vi "rszvl_core_global.vi"() -> ()   [LabVIEW 2014] (continued)
Callback"="", "Coerce Callback"="", "User Callback"="", "Supported Models"="", "Instrument Options"="", "Repeated Capabilities"="", "Restricted Repeated Capabilities"="", "Help"="This attribute defines an absolute threshold value for limit lines with relative Y axis scaling. The absolute threshold value is used in the limit check as soon as it exceeds the relative limit value.\n\nAvailable Repeated Capabilities:\nLimit: L1,L2,L3,L4,L5,L6,L7,L8\r\n\nRemote-control command(s):\nCALCulate<1|2>:LIMit<1 to 8>:LOWer:THReshold", "Flags"={"OPC Wait"=FALSE, "Dont check status"=FALSE, "*WAI"=FALSE}, "Check Status Callback"=""}, {"Level"=3, "Descriptive Name"="Limit Line Lower Offset", "Class Only"=FALSE, "Data Type"=1, "Access"=2, "Identifier"="RSZVL_LIMIT_LOWER_OFFSET", "Range Table"="rszvl_rngRefLevel", "Command"="CALC:LIM{Limit}:LOW:OFFS", "Read Callback"="", "Write Callback"="", "Range Callback"="", "Check Callback"="", "Rngtable Callback"="", "Coerce Callback"="", "User Callback"="", "Supported Models"="", "Instrument Options"="", "Repeated Capabilities"="", "Restricted Repeated Capabilities"="", "Help"="This attribute defines an offset for the Y axis of the selected relative lower limit line. In contrast to SHIF, the line is not shifted by modifying the individual Y values but by means of an additive offset.\n\nAvailable Repeated Capabilities:\nLimit: L1,L2,L3,L4,L5,L6,L7,L8\r\n\nRemote-control command(s):\nCALCulate<1|2>:LIMit<1 to 8>:LOWer:OFFSet", "Flags"={"OPC Wait"=FALSE, "Dont check status"=FALSE, "*WAI"=FALSE}, "Check Status Callback"=""}, {"Level"=3, "Descriptive Name"="Limit Line Lower Shift", "Class Only"=FALSE, "Data Type"=1, "Access"=1, "Identifier"="RSZVL_LIMIT_LOWER_SHIFT", "Range Table"="rszvl_rngLimitOffset", "Command"="CALC:LIM{Limit}:LOW:SHIF", "Read Callback"="", "Write Callback"="", "Range Callback"="", "Check Callback"="", "Rngtable Callback"="", "Coerce Callback"="", "User Callback"="", "Supported Models"="", "Instrument Options"="", "Repeated Capabilities"="", "Restricted Repeated Capabilities"="", "Help"="This attribute shifts a limit line by the indicated value in Y direction. In contrast to offset, the line is shifted by modifying the individual Y values but not by means of an additive offset.\n\nAvailable Repeated Capabilities:\nLimit: L1,L2,L3,L4,L5,L6,L7,L8\r\n\nRemote-control command(s):\nCALCulate<1|2>:LIMit<1 to 8>:LOWer:SHIFt", "Flags"={"OPC Wait"=FALSE, "Dont check status"=FALSE, "*WAI"=FALSE}, "Check Status Callback"=""}, {"Level"=2, "Descriptive Name"="Upper Limit", "Class Only"=TRUE, "Data Type"=0, "Access"=0, "Identifier"="", "Range Table"="", "Command"="", "Read Callback"="", "Write Callback"="", "Range Callback"="", "Check Callback"="", "Rngtable Callback"="", "Coerce Callback"="", "User Callback"="", "Supported Models"="", "Instrument Options"="", "Repeated Capabilities"="", "Restricted Repeated Capabilities"="", "Help"="(1) Limit Line Upper State:\nThis attribute switches on or off the indicated limit line.\n\n(2) Limit Line Upper Scaling:\nThis command selects the relative or absolute scaling for the Y axis of the selected upper limit line. Selecting RELative causes the unit to be switched to DB.\n\n(3) Limit Line Upper Spacing:\nThis attribute selects linear or logarithmic interpolation for the upper limit line.\n\n(4) Limit Line Upper Margin:\nThis attribute defines a margin to an upper limit line, at which out-of-limit values are signalled (if the limit check is active), but not handled as a violation of the limit value.\n\n(5) Limit Line Upper Threshold:\nThis attribute defines an absolute threshold value for limit lines with relative Y axis scaling. The absolute threshold value is used in the limit check as soon as it exceeds the relative limit value.\n\n(6) Limit Line Upper Offset:\nThis attribute defines an offset for the Y axis of the selected relative upper limit line. In contrast to shift, the line is not shifted by modifying the individual Y values but by means of an additive offset.\n\n(7) Limit Line Upper Shift:\nThis attribute moves a limit line by the indicated value in Y direction. In contrast to offset, the line is shifted by modifying the individual Y values and not by means of an additive offset.", "Flags"={"OPC Wait"=FALSE, "Dont check status"=FALSE, "*WAI"=FALSE}, "Check Status Callback"=""}, {"Level"=3, "Descriptive Name"="Limit Line Upper State", "Class Only"=FALSE, "Data Type"=3, "Access"=2, "Identifier"="RSZVL_LIMIT_UPPER_STATE", "Range Table"="", "Command"="CALC:LIM{Limit}:UPP:STAT", "Read Callback"="", "Write Callback"="", "Range Callback"="", "Check Callback"="", "Rngtable Callback"="", "Coerce Callback"="", "User Callback"="", "Supported Models"="", "Instrument Options"="", "Repeated Capabilities"="", "Restricted Repeated Capabilities"="", "Help"="This attribute switches on or off the indicated limit line.\n\nAvailable Repeated Capabilities:\nLimit: L1,L2,L3,L4,L5,L6,L7,L8\r\n\nRemote-control command(s):\nCALCulate<1|2>:LIMit<1 to 8>:UPPer:STATe ON | OFF", "Flags"={"OPC Wait"=FALSE, "Dont check status"=FALSE, "*WAI"=FALSE}, "Check Status Callback"=""}, {"Level"=3, "Descriptive Name"="Limit Line Upper Scaling", "Class Only"=FALSE, "Data Type"=0, "Access"=2, "Identifier"="RSZVL_LIMIT_UPPER_SCALING", "Range Table"="rszvl_rngAbsRel", "Command"="CALC:LIM{Limit}:UPP:MODE", "Read Callback"="", "Write Callback"="", "Range Callback"="", "Check Callback"="", "Rngtable Callback"="", "Coerce Callback"="", "User Callback"="", "Supported Models"="", "Instrument Options"="", "Repeated Capabilities"="", "Restricted Repeated Capabilities"="", "Help"="This command selects the relative or absolute scaling for the Y axis of the selected upper limit line. Selecting RELative causes the unit to be switched to DB.\n\nAvailable Repeated Capabilities:\nLimit: L1,L2,L3,L4,L5,L6,L7,L8\r\n\nRemote-control command(s):\nCALCulate<1|2>:LIMit<1 to 8>:UPPer:MODE RELative | ABSolute", "Flags"={"OPC Wait"=FALSE, "Dont check status"=FALSE, "*WAI"=FALSE}, "Check Status Callback"=""}, {"Level"=3, "Descriptive Name"="Limit Line Upper Spacing", "Class Only"=FALSE, "Data Type"=0, "Access"=2, "Identifier"="RSZVL_LIMIT_UPPER_SPACING", "Range Table"="rszvl_rngLinLog", "Command"="CALC:LIM{Limit}:UPP:SPAC", "Read Callback"="", "Write Callback"="", "Range Callback"="", "Check Callback"="", "Rngtable Callback"="", "Coerce Callback"="", "User Callback"="", "Supported Models"="", "Instrument Options"="", "Repeated Capabilities"="", "Restricted Repeated Capabilities"="", "Help"="This attribute selects linear or logarithmic interpolation for the upper limit line.\n\nAvailable Repeated Capabilities:\nLimit: L1,L2,L3,L4,L5,L6,L7,L8\r\n\nRemote-control command(s):\nCALCulate<1|2>:LIMit<1 to 8>:UPPer:SPACing LINear | LOGarithmic", "Flags"={"OPC Wait"=FALSE, "Dont check status"=FALSE, "*WAI"=FALSE}, "Check Status Callback"=""}, {"Level"=3, "Descriptive Name"="Limit Line Upper Margin", "Class Only"=FALSE, "Data Type"=1, "Access"=2, "Identifier"="RSZVL_LIMIT_UPPER_MARGIN", "Range Table"="rszvl_rngLimitMargin", "Command"="CALC:LIM{Limit}:UPP:MARG", "Read Callback"="", "Write Callback"="", "Range Callback"="", "Check Callback"="", "Rngtable Callback"="", "Coerce Callback"="", "User Callback"="", "Supported Models"="", "Instrument Options"="", "Repeated Capabilities"="", "Restricted Repeated Capabilities"="", "Help"="This attribute defines a margin to an upper limit line, at which out-of-limit values are signalled (if the limit check is active), but not handled as a violation of the limit value.\n\nAvailable Repeated Capabilities:\nLimit: L1,L2,L3,L4,L5,L6,L7,L8\r\n\nRemote-control command(s):\nCALCulate<1|2>:LIMit<1 to 8>:UPPer:MARGin", "Flags"={"OPC Wait"=FALSE, "Dont check status"=FALSE, "*WAI"=FALSE}, "Check Status Callback"=""}, {"Level"=3, "Descriptive Name"="Limit Line Upper Threshold", "Class Only"=FALSE, "Data Type"=1, "Access"=2, "Identifier"="RSZVL_LIMIT_UPPER_THRESHOLD", "Range Table"="rszvl_rngRefLevel", "Command"="CALC:LIM{Limit}:UPP:THR", "Read Callback"="", "Write Callback"="", "Range Callback"="", "Check Callback"="", "Rngtable Callback"="", "Coerce Callback"="", "User Callback"="", "Supported Models"="", "Instrument Options"="", "Repeated Capabilities"="", "Restricted Repeated Capabilities"="", "Help"="This attribute defines an absolute threshold value for limit lines with relative Y axis scaling. The absolute threshold value is used in the limit check as soon as it exceeds the relative limit value.\n\nAvailable Repeated Capabilities:\nLimit: L1,L2,L3,L4,L5,L6,L7,L8\r\n\nRemote-control command(s):\nCALCulate<1|2>:LIMit<1 to 8>:UPPer:THReshold", "Flags"={"OPC Wait"=FALSE, "Dont check status"=FALSE, "*WAI"=FALSE}, "Check Status Callback"=""}, {"Level"=3, "Descriptive Name"="Limit Line Upper Offset", "Class Only"=FALSE, "Data Type"=1, "Access"=2, "Identifier"="RSZVL_LIMIT_UPPER_OFFSET", "Range Table"="rszvl_rngRefLevel", "Command"="CALC:LIM{Limit}:UPP:OFFS", "Read Callback"="", "Write Callback"="", "Range Callback"="", "Check Callback"="", "Rngtable Callback"="", "Coerce Callback"="", "User Callback"="", "Supported Models"="", "Instrument Options"="", "Repeated Capabilities"="", "Restricted Repeated Capabilities"="", "Help"="This attribute defines an offset for the Y axis of the selected relative upper limit line. In contrast to shift, the line is not shifted by modifying the individual Y values but by means of an additive offset.\n\nAvailable Repeated Capabilities:\nLimit: L1,L2,L3,L4,L5,L6,L7,L8\r\n\nRemote-control command(s):\nCALCulate<1|2>:LIMit<1 to 8>:UPPer:OFFSet", "Flags"={"OPC Wait"=FALSE, "Dont check status"=FALSE, "*WAI"=FALSE}, "Check Status Callback"=""}, {"Level"=3, "Descriptive Name"="Limit Line Upper Shift", "Class Only"=FALSE, "Data Type"=1, "Access"=1, "Identifier"="RSZVL_LIMIT_UPPER_SHIFT", "Range Table"="rszvl_rngLimitOffset", "Command"="CALC:LIM{Limit}:UPP:SHIF", "Read Callback"="", "Write Callback"="", "Range Callback"="", "Check Callback"="", "Rngtable Callback"="", "Coerce Callback"="", "User Callback"="", "Supported Models"="", "Instrument Options"="", "Repeated Capabilities"="", "Restricted Repeated Capabilities"="", "Help"="This attribute moves a limit line by the indicated value in Y direction. In contrast to offset, the line is shifted by modifying the individual Y values and not by means of an additive offset.\n\nAvailable Repeated Capabilities:\nLimit: L1,L2,L3,L4,L5,L6,L7,L8\r\n\nRemote-control command(s):\nCALCulate<1|2>:LIMit<1 to 8>:UPPer:SHIFt", "Flags"={"OPC Wait"=FALSE, "Dont check status"=FALSE, "*WAI"=FALSE}, "Check Status Callback"=""}, {"Level"=2, "Descriptive Name"="Display Lines", "Class Only"=TRUE, "Data Type"=0, "Access"=0, "Identifier"="", "Range Table"="", "Command"="", "Read Callback"="", "Write Callback"="", "Range Callback"="", "Check Callback"="", "Rngtable Callback"="", "Coerce Callback"="", "User Callback"="", "Supported Models"="", "Instrument Options"="", "Repeated Capabilities"="", "Restricted Repeated Capabilities"="", "Help"="(1) Threshold Line State:\nThis attribute switches on or off the threshold line.\n\n(2) Threshold Line Position:\nThis attribute defines the threshold value for the maximum/minimum search of markers with marker search functions MAX PEAK, NEXT PEAK, etc.\n\n(3) Display Line State:\nThis attribute switches Display Line 1 or 2 (level lines) on or off.\n\n(4) Display Line Position:\nThis attribute defines the position of Display Line 1 or 2. These lines enable the user to mark any levels in the diagram. The unit depends on the setting made with CALC:UNIT.\n\n(5) Frequency Line State:\nThis attribute switches the frequency line on or off.\n\n(6) Frequency Line Position:\nThis attribute defines the position of the frequency lines.\nThe frequency lines mark the frequencies. Frequency lines are only available with SPAN > 0.\n\n(7) Time Line State:\nThis attribute switches the time line on or off.\n\n(8) Time Line Position:\nThis attribute defines the position of the time lines.\nThe time lines mark the times. Time lines are only available with SPAN = 0.", "Flags"={"OPC Wait"=FALSE, "Dont check status"=FALSE, "*WAI"=FALSE}, "Check Status Callback"=""}, {"Level"=3, "Descriptive Name"="Threshold Line State", "Class Only"=FALSE, "Data Type"=3, "Access"=2, "Identifier"="RSZVL_ATTR_THRLINE_STATE", "Range Table"="", "Command"="CALC:THR:STAT", "Read Callback"="", "Write Callback"="", "Range Callback"="", "Check Callback"="", "Rngtable Callback"="", "Coerce Callback"="", "User Callback"="", "Supported Models"="", "Instrument Options"="", "Repeated Capabilities"="", "Restricted Repeated Capabilities"="", "Help"="This attribute switches on or off the threshold line.\n\nAvailable Repeated Capabilities:\nNone\n\nRemote-control command(s):\nCALCulate<1|2>:THReshold:STATe ON | OFF", "Flags"={"OPC Wait"=FALSE, "Dont check status"=FALSE, "*WAI"=FALSE}, "Check Status Callback"=""}, {"Level"=3, "Descriptive Name"="Threshold Line Position", "Class Only"=FALSE, "Data Type"=1, "Access"=2, "Identifier"="RSZVL_ATTR_THRLINE_POSITION", "Range Table"="", "Command"="CALC:THR", "Read Callback"="", "Write Callback"="", "Range Callback"="", "Check Callback"="", "Rngtable Callback"="", "Coerce Callback"="", "User Callback"="", "Supported Models"="", "Instrument Options"="", "Repeated Capabilities"="", "Restricted Repeated Capabilities"="", "Help"="This attribute defines the threshold value for the maximum/minimum search of markers with marker search functions MAX PEAK, NEXT PEAK, etc.\n\nAvailable Repeated Capabilities:\nNone\n\nRemote-control command(s):\nCALCulate<1|2>:THReshold", "Flags"={"OPC Wait"=FALSE, "Dont check status"=FALSE, "*WAI"=FALSE}, "Check Status Callback"=""}, {"Level"=3, "Descriptive Name"="Display Line State", "Class Only"=FALSE, "Data Type"=3, "Access"=2, "Identifier"="RSZVL_ATTR_DLINE_STATE", "Range Table"="", "Command"="CALC:DLIN{Line}:STAT", "Read Callback"="", "Write Callback"="", "Range Callback"="", "Check Callback"="", "Rngtable Callback"="", "Coerce Callback"="", "User Callback"="", "Supported Models"="", "Instrument Options"="", "Repeated Capabilities"="", "Restricted Repeated Capabilities"="", "Help"="This attribute switches Display Line 1 or 2 (level lines) on or off.\n\nAvailable Repeated Capabilities:\nLine: L1,L2\r\n\nRemote-control command(s):\nCALCulate<1|2>:DLINe<1|2>:STATe ON | OFF", "Flags"={"OPC Wait"=FALSE, "Dont check status"=FALSE, "*WAI"=FALSE}, "Check Status Callback"=""}, {"Level"=3, "Descriptive Name"="Display Line Position", "Class Only"=FALSE, "Data Type"=1, "Access"=2, "Identifier"="RSZVL_ATTR_DLINE_POSITION", "Range Table"="", "Command"="CALC:DLIN{Line}", "Read Callback"="", "Write Callback"="", "Range Callback"="", "Check Callback"="", "Rngtable Callback"="", "Coerce Callback"="", "User Callback"="", "Supported Models"="", "Instrument Options"="", "Repeated Capabilities"="", "Restricted Repeated Capabilities"="", "Help"="This attribute defines the position of Display Line 1 or 2. These lines enable the user to mark any levels in the diagram. The unit depends on the setting made with CALC:UNIT.\n\nAvailable Repeated Capabilities:\nLine: L1,L2\r\n\nRemote-control command(s):\nCALCulate<1|2>:DLINe<1|2>", "Flags"={"OPC Wait"=FALSE, "Dont check status"=FALSE, "*WAI"=FALSE}, "Check Status Callback"=""}, {"Level"=3, "Descriptive Name"="Frequency Line State", "Class Only"=FALSE, "Data Type"=3, "Access"=2, "Identifier"="RSZVL_ATTR_FLINE_STATE", "Range Table"="", "Command"="CALC:FLIN{Line}:STAT", "Read Callback"="", "Write Callback"="", "Range Callback"="", "Check Callback"="", "Rngtable Callback"="", "Coerce Callback"="", "User Callback"="", "Supported Models"="", "Instrument Options"="", "Repeated Capabilities"="", "Restricted Repeated Capabilities"="", "Help"="This attribute switches the frequency line on or off.\n\nAvailable Repeated Capabilities:\nLine: L1,L2\r\n\nRemote-control command(s):\nCALCulate<1|2>:FLINe<1|2>:STATe ON | OFF", "Flags"={"OPC Wait"=FALSE, "Dont check status"=FALSE, "*WAI"=FALSE}, "Check Status Callback"=""}, {"Level"=3, "Descriptive Name"="Frequency Line Position", "Class Only"=FALSE, "Data Type"=1, "Access"=2, "Identifier"="RSZVL_ATTR_FLINE_POSITION", "Range Table"="", "Command"="CALC:FLIN{Line}", "Read Callback"="", "Write Callback"="", "Range Callback"="", "Check Callback"="", "Rngtable Callback"="", "Coerce Callback"="", "User Callback"="", "Supported Models"="", "Instrument Options"="", "Repeated Capabilities"="", "Restricted Repeated Capabilities"="", "Help"="This attribute defines the position of the frequency lines.\nThe frequency lines mark the frequencies. Frequency lines are only available with SPAN > 0.\n\nAvailable Repeated Capabilities:\nLine: L1,L2\r\n\nRemote-control command(s):\nCALCulate<1|2>:FLINe<1|2>", "Flags"={"OPC Wait"=FALSE, "Dont check status"=FALSE, "*WAI"=FALSE}, "Check Status Callback"=""}, {"Level"=3, "Descriptive Name"="Time Line State", "Class Only"=FALSE, "Data Type"=3, "Access"=2, "Identifier"="RSZVL_ATTR_TLINE_STATE", "Range Table"="", "Command"="CALC:TLIN{Line}:STAT", "Read Callback"="", "Write Callback"="", "Range Callback"="", "Check Callback"="", "Rngtable Callback"="", "Coerce Callback"="", "User Callback"="", "Supported Models"="", "Instrument Options"="", "Repeated Capabilities"="", "Restricted Repeated Capabilities"="", "Help"="This attribute switches the time line on or off.\n\nAvailable Repeated Capabilities:\nLine: L1,L2\r\n\nRemote-control command(s):\nCALCulate<1|2>:TLINe<1|2>:STATe ON | OFF", "Flags"={"OPC Wait"=FALSE, "Dont check status"=FALSE, "*WAI"=FALSE}, "Check Status Callback"=""}, {"Level"=3, "Descriptive Name"="Time Line Position", "Class Only"=FALSE, "Data Type"=1, "Access"=2, "Identifier"="RSZVL_ATTR_TLINE_POSITION", "Range Table"="rszvl_rngTimeLinePos", "Command"="CALC:TLIN{Line}", "Read Callback"="", "Write Callback"="", "Range Callback"="", "Check Callback"="", "Rngtable Callback"="", "Coerce Callback"="", "User Callback"="", "Supported Models"="", "Instrument Options"="", "Repeated Capabilities"="", "Restricted Repeated Capabilities"="", "Help"="This attribute defines the position of the time lines.\nThe time lines mark the times. Time lines are only available with SPAN = 0.\n\nAvailable Repeated Capabilities:\nLine: L1,L2\r\n\nRemote-control command(s):\nCALCulate<1|2>:TLINe<1|2>", "Flags"={"OPC Wait"=FALSE, "Dont check status"=FALSE, "*WAI"=FALSE}, "Check Status Callback"=""}, {"Level"=1, "Descriptive Name"="Trigger", "Class Only"=TRUE, "Data Type"=0, "Access"=0, "Identifier"="", "Range Table"="", "Command"="", "Read Callback"="", "Write Callback"="", "Range Callback"="", "Check Callback"="", "Rngtable Callback"="", "Coerce Callback"="", "User Callback"="", "Supported Models"="", "Instrument Options"="", "Repeated Capabilities"="", "Restricted Repeated Capabilities"="", "Help"="(1) Trigger Source:\nThis attribute selects the trigger source for the start of a sweep.\n\n(2) Trigger Delay:\nThis attribute defines the length of the trigger delay.\n\nNote:\n(1) A negative delay time (pretrigger) can be set in the time domain (span < 0 Hz) only.\n\n(3) Trigger Slope:\nThis attribute selects the slope of the trigger signal. The selected trigger slope applies to all trigger signal sources .\n\n(4) External Trigger (Class):\nAttributes to configure and control external triggers.\n\n(1) External Gate:\nThis attribute switches on/off the sweep control by an external gate signal. If the external gate is selected the trigger source is automatically switched to EXTernal as well. \nIn case of measurement with external gate, the measured values are recorded as long as the gate is opened. There are two possibilities:\n\n1. The gate is edge-triggered (SWEep:EGATe:TYPE EDGE): After detection of the set gate signal edge, the gate remains open until the gate delay (SWEep:EGATe:HOLDoff) has expired.\n\n2. The gate is level-triggered (SWEep:EGATe:TYPE LEVel): After detection of the gate signal, the gate remains open until the gate signal disappears.\n\nA delay between applying the gate signal and the start of recording measured values can be defined\nwith SWEep:EGATe:HOLDoff.\nDuring a sweep the gate can be opened and closed several times. The synchronization mechanisms\nwith *OPC, *OPC? and *WAI remain completely unaffected.\nThe sweep end is detected when the required number of measurement points (625 in analyzer\nmode) has been recorded.\n\nNote: \n(1) This attribute is not available for GSM/EDGE measurements modulation accuracy (MAC),\nphase/frequency error (PFE), power versus time (PVT ), carrier power (CPW), spectrum\ndue to switching (TRA) and spurious emissions (SPU).\n\n(2) External Gate Delay:\nThis attribute defines the delay time between the external gate signal and the continuation of the sweep.\n\n(3) External Gate Mode:\nThis attribute sets the type of triggering (level or edge) by the external gate signal.\nThe gate opening time cannot be defined with the parameter EGATe:LENGth in case of level triggering. The gate is closed when the gate signal disappears.\n\n(4) External Gate Polarity:\nThis attribute determines the polarity of the external gate signal. The setting is valid both for the edge of an edge-triggered signal and the level of a level-triggered signal.\n\n(5) External Gate Length:\nThis attribute determines the time interval during which the instrument sweeps.\n\n(6) External Gate Signal Source:\nThis attribute toggles between external gate signal and IF power signal as a signal source for the gate mode. If an IF power signal is used, the gate is opened as soon as a signal at > -20 dBm is detected within the IF path bandwidth (50 MHz).\n\n\n\n(5) Video Trigger (Class):\nAttributes to configure and control video triggers.\n\n(1) Video Trigger Level:\nThis attribute sets the level of the video trigger source.\n\n\n\n(6) IF Power Trigger (Class):\nIF Power Trigger configuration.\n\n(1) Trigger IF Power Level:\nThis attribute sets the level of the IF power trigger source.\n\n(2) Trigger IF Power Offset:\nThis attribute sets the holding time before the next IF power trigger event.\n\n(3) Trigger IF Power Hysteresis:\nThis attribute sets the limit that the hysteresis value has to fall below in order to trigger the next measurement.\n\n\n\n(7) Time Trigger (Class):\nTime Trigger configuration.\n\n(1) Time Interval:\nThis attribute sets the time intervall for the time trigger source.", "Flags"={"OPC Wait"=FALSE, "Dont check status"=FALSE, "*WAI"=FALSE}, "Check Status Callback"=""}, {"Level"=2, "Descriptive Name"="Trigger Source", "Class Only"=FALSE, "Data Type"=0, "Access"=2, "Identifier"="RSZVL_ATTR_TRIGGER_SOURCE", "Range Table"="rszvl_rngTriggerSource", "Command"="TRIG{Channel}:SOUR", "Read Callback"="", "Write Callback"="", "Range Callback"="", "Check Callback"="", "Rngtable Callback"="", "Coerce Callback"="", "User Callback"="", "Supported Models"="", "Instrument Options"="", "Repeated Capabilities"="", "Restricted Repeated Capabilities"="", "Help"="This attribute selects the trigger source for the start of a sweep.\n\nAvailable Repeated Capabilities:\nChannel: CH1,CH2,CH3,CH4,CH5,CH6,CH7,CH8,CH9,CH10,CH11,CH12,CH13,CH14,CH15,CH16,CH17,CH18,CH19,CH20\r\n\nRemote-control command(s):\nTRIGger<Channel>[:SEQuence]:SOURce", "Flags"={"OPC Wait"=FALSE, "Dont check status"=FALSE, "*WAI"=FALSE}, "Check Status Callback"=""}, {"Level"=2, "Descriptive Name"="Trigger Delay", "Class Only"=FALSE, "Data Type"=1, "Access"=2, "Identifier"="RSZVL_ATTR_TRIGGER_DELAY", "Range Table"="rszvl_rngTriggerDelay", "Command"="TRIG{Channel}:HOLD", "Read Callback"="", "Write Callback"="", "Range Callback"="", "Check Callback"="", "Rngtable Callback"="", "Coerce Callback"="", "User Callback"="", "Supported Models"="", "Instrument Options"="", "Repeated Capabilities"="", "Restricted Repeated Capabilities"="", "Help"="This attribute defines the length of the trigger delay.\n\nNote:\n(1) A negative delay time (pretrigger) can be set in the time domain (span < 0 Hz) only.\n\nAvailable Repeated Capabilities:\nChannel: CH1,CH2,CH3,CH4,CH5,CH6,CH7,CH8,CH9,CH10,CH11,CH12,CH13,CH14,CH15,CH16,CH17,CH18,CH19,CH20\r\n\nRemote-control command(s):\nTRIGger<Channel>[:SEQuence]:HOLDoff", "Flags"={"OPC Wait"=FALSE, "Dont check status"=FALSE, "*WAI"=FALSE}, "Check Status Callback"=""}, {"Level"=2, "Descriptive Name"="Trigger Slope", "Class Only"=FALSE, "Data Type"=0, "Access"=2, "Identifier"="RSZVL_ATTR_TRIGGER_SLOPE", "Range Table"="rszvl_rngPolarity", "Command"="TRIG{Channel}:SLOP", "Read Callback"="", "Write Callback"="", "Range Callback"="", "Check Callback"="", "Rngtable Callback"="", "Coerce Callback"="", "User Callback"="", "Supported Models"="", "Instrument Options"="", "Repeated Capabilities"="", "Restricted Repeated Capabilities"="", "Help"="This attribute selects the slope of the trigger signal. The selected trigger slope applies to all trigger signal sources .\n\nAvailable Repeated Capabilities:\nChannel: CH1,CH2,CH3,CH4,CH5,CH6,CH7,CH8,CH9,CH10,CH11,CH12,CH13,CH14,CH15,CH16,CH17,CH18,CH19,CH20\r\n\nRemote-control command(s):\nTRIGger<Channel>[:SEQuence]:SLOPe POSitive | NEGative", "Flags"={"OPC Wait"=FALSE, "Dont check status"=FALSE, "*WAI"=FALSE}, "Check Status Callback"=""}, {"Level"=2, "Descriptive Name"="Trigger Event Start", "Class Only"=FALSE, "Data Type"=0, "Access"=2, "Identifier"="RSZVL_ATTR_TRIGGER_EVENT_START", "Range Table"="rszvl_rngEventStart", "Command"="TRIG{Channel}:LINK", "Read Callback"="", "Write Callback"="", "Range Callback"="", "Check Callback"="", "Rngtable Callback"="", "Coerce Callback"="", "User Callback"="", "Supported Models"="", "Instrument Options"="", "Repeated Capabilities"="", "Restricted Repeated Capabilities"="", "Help"="Selects the Triggered Meas. Sequence. The identifier for the sequence is a string variable.\n\nAvailable Repeated Capabilities:\nChannel: CH1,CH2,CH3,CH4,CH5,CH6,CH7,CH8,CH9,CH10,CH11,CH12,CH13,CH14,CH15,CH16,CH17,CH18,CH19,CH20\r\n\nRemote-control command(s):\nTRIGger<Ch>[:SEQuence]:LINK 'POINt' | 'SWEep'", "Flags"={"OPC Wait"=FALSE, "Dont check status"=FALSE, "*WAI"=FALSE}, "Check Status Callback"=""}, {"Level"=2, "Descriptive Name"="External Trigger", "Class Only"=TRUE, "Data Type"=0, "Access"=0, "Identifier"="", "Range Table"="", "Command"="", "Read Callback"="", "Write Callback"="", "Range Callback"="", "Check Callback"="", "Rngtable Callback"="", "Coerce Callback"="", "User Callback"="", "Supported Models"="", "Instrument Options"="", "Repeated Capabilities"="", "Restricted Repeated Capabilities"="", "Help"="Attributes to configure and control external triggers.\n\n(1) External Gate:\nThis attribute switches on/off the sweep control by an external gate signal. If the external gate is selected the trigger source is automatically switched to EXTernal as well. \nIn case of measurement with external gate, the measured values are recorded as long as the gate is opened. There are two possibilities:\n\n1. The gate is edge-triggered (SWEep:EGATe:TYPE EDGE): After detection of the set gate signal edge, the gate remains open until the gate delay (SWEep:EGATe:HOLDoff) has expired.\n\n2. The gate is level-triggered (SWEep:EGATe:TYPE LEVel): After detection of the gate signal, the gate remains open until the gate signal disappears.\n\nA delay between applying the gate signal and the start of recording measured values can be defined\nwith SWEep:EGATe:HOLDoff.\nDuring a sweep the gate can be opened and closed several times. The synchronization mechanisms\nwith *OPC, *OPC? and *WAI remain completely unaffected.\nThe sweep end is detected when the required number of measurement points (625 in analyzer\nmode) has been recorded.\n\nNote: \n(1) This attribute is not available for GSM/EDGE measurements modulation accuracy (MAC),\nphase/frequency error (PFE), power versus time (PVT ), carrier power (CPW), spectrum\ndue to switching (TRA) and spurious emissions (SPU).\n\n(2) External Gate Delay:\nThis attribute defines the delay time between the external gate signal and the continuation of the sweep.\n\n(3) External Gate Mode:\nThis attribute sets the type of triggering (level or edge) by the external gate signal.\nThe gate opening time cannot be defined with the parameter EGATe:LENGth in case of level triggering. The gate is closed when the gate signal disappears.\n\n(4) External Gate Polarity:\nThis attribute determines the polarity of the external gate signal. The setting is valid both for the edge of an edge-triggered signal and the level of a level-triggered signal.\n\n(5) External Gate Length:\nThis attribute determines the time interval during which the instrument sweeps.\n\n(6) External Gate Signal Source:\nThis attribute toggles between external gate signal and IF power signal as a signal source for the gate mode. If an IF power signal is used, the gate is opened as soon as a signal at > -20 dBm is detected within the IF path bandwidth (50 MHz).", "Flags"={"OPC Wait"=FALSE, "Dont check status"=FALSE, "*WAI"=FALSE}, "Check Status Callback"=""}, {"Level"=3, "Descriptive Name"="External Gate", "Class Only"=FALSE, "Data Type"=3, "Access"=2, "Identifier"="RSZVL_ATTR_EXTERNAL_GATE", "Range Table"="", "Command"="SENS:SWE:EGAT", "Read Callback"="", "Write Callback"="", "Range Callback"="", "Check Callback"="", "Rngtable Callback"="", "Coerce Callback"="", "User Callback"="", "Supported Models"="", "Instrument Options"="", "Repeated Capabilities"="", "Restricted Repeated Capabilities"="", "Help"="This attribute switches on/off the sweep control by an external gate signal. If the external gate is selected the trigger source is automatically switched to EXTernal as well. \nIn case of measurement with external gate, the measured values are recorded as long as the gate is opened. There are two possibilities:\n\n1. The gate is edge-triggered (SWEep:EGATe:TYPE EDGE): After detection of the set gate signal edge, the gate remains open until the gate delay (SWEep:EGATe:HOLDoff) has expired.\n\n2. The gate is level-triggered (SWEep:EGATe:TYPE LEVel): After detection of the gate signal, the gate remains open until the gate signal disappears.\n\nA delay between applying the gate signal and the start of recording measured values can be defined\nwith SWEep:EGATe:HOLDoff.\nDuring a sweep the gate can be opened and closed several times. The synchronization mechanisms\nwith *OPC, *OPC? and *WAI remain completely unaffected.\nThe sweep end is detected when the required number of measurement points (625 in analyzer\nmode) has been recorded.\n\nNote: \n(1) This attribute is not available for GSM/EDGE measurements modulation accuracy (MAC),\nphase/frequency error (PFE), power versus time (PVT ), carrier power (CPW), spectrum\ndue to switching (TRA) and spurious emissions (SPU).\n\nAvailable Repeated Capabilities:\nNone\n\nRemote-control command(s):\n[SENSe<1|2>:]SWEep:EGATe ON | OFF", "Flags"={"OPC Wait"=FALSE, "Dont check status"=FALSE, "*WAI"=FALSE}, "Check Status Callback"=""}, {"Level"=3, "Descriptive Name"="External Gate Delay", "Class Only"=FALSE, "Data Type"=1, "Access"=2, "Identifier"="RSZVL_ATTR_EXTERNAL_GATE_HOLD", "Range Table"="rszvl_rngExtGateDelay", "Command"="SENS:SWE:EGAT:HOLD", "Read Callback"="", "Write Callback"="", "Range Callback"="", "Check Callback"="", "Rngtable Callback"="", "Coerce Callback"="", "User Callback"="", "Supported Models"="", "Instrument Options"="", "Repeated Capabilities"="", "Restricted Repeated Capabilities"="", "Help"="This attribute defines the delay time between the external gate signal and the continuation of the sweep.\n\nAvailable Repeated Capabilities:\nNone\n\nRemote-control command(s):\n[SENSe<1|2>:]SWEep:EGATe:HOLDoff", "Flags"={"OPC Wait"=FALSE, "Dont check status"=FALSE, "*WAI"=FALSE}, "Check Status Callback"=""}, {"Level"=3, "Descriptive Name"="External Gate Mode", "Class Only"=FALSE, "Data Type"=0, "Access"=2, "Identifier"="RSZVL_ATTR_EXTERNAL_GATE_TRIGGER_TYPE", "Range Table"="rszvl_rngExtGateTrigType", "Command"="SENS:SWE:EGAT:TYPE", "Read Callback"="", "Write Callback"="", "Range Callback"="", "Check Callback"="", "Rngtable Callback"="", "Coerce Callback"="", "User Callback"="", "Supported Models"="", "Instrument Options"="", "Repeated Capabilities"="", "Restricted Repeated Capabilities"="", "Help"="This attribute sets the type of triggering (level or edge) by the external gate signal.\nThe gate opening time cannot be defined with the parameter EGATe:LENGth in case of level triggering. The gate is closed when the gate signal disappears.\n\nAvailable Repeated Capabilities:\nNone\n\nRemote-control command(s):\n[SENSe<1|2>:]SWEep:EGATe:TYPE LEVel | EDGE", "Flags"={"OPC Wait"=FALSE, "Dont check status"=FALSE, "*WAI"=FALSE}, "Check Status Callback"=""}, {"Level"=3, "Descriptive Name"="External Gate Polarity", "Class Only"=FALSE, "Data Type"=0, "Access"=2, "Identifier"="RSZVL_ATTR_EXTERNAL_GATE_POLARITY", "Range Table"="rszvl_rngPolarity", "Command"="SENS:SWE:EGATe:POL", "Read Callback"="", "Write Callback"="", "Range Callback"="", "Check Callback"="", "Rngtable Callback"="", "Coerce Callback"="", "User Callback"="", "Supported Models"="", "Instrument Options"="", "Repeated Capabilities"="", "Restricted Repeated Capabilities"="", "Help"="This attribute determines the polarity of the external gate signal. The setting is valid both for the edge of an edge-triggered signal and the level of a level-triggered signal.\n\nAvailable Repeated Capabilities:\nNone\n\nRemote-control command(s):\n[SENSe<1|2>:]SWEep:EGATe:POLarity POSitive | NEGative", "Flags"={"OPC Wait"=FALSE, "Dont check status"=FALSE, "*WAI"=FALSE}, "Check Status Callback"=""}, {"Level"=3, "Descriptive Name"="External Gate Length", "Class Only"=FALSE, "Data Type"=1, "Access"=2, "Identifier"="RSZVL_ATTR_EXTERNAL_GATE_LENGTH", "Range Table"="rszvl_rngExtGateLength", "Command"="SENS:SWE:EGAT:LENG", "Read Callback"="", "Write Callback"="", "Range Callback"="", "Check Callback"="", "Rngtable Callback"="", "Coerce Callback"="", "User Callback"="", "Supported Models"="", "Instrument Options"="", "Repeated Capabilities"="", "Restricted Repeated Capabilities"="", "Help"="This attribute determines the time interval during which the instrument sweeps.\n\nAvailable Repeated Capabilities:\nNone\n\nRemote-control command(s):\n[SENSe<1|2>:]SWEep:EGATe:LENGth", "Flags"={"OPC Wait"=FALSE, "Dont check status"=FALSE, "*WAI"=FALSE}, "Check Status Callback"=""}, {"Level"=3, "Descriptive Name"="External Gate Signal Source", "Class Only"=FALSE, "Data Type"=0, "Access"=2, "Identifier"="RSZVL_ATTR_EXTERNAL_GATE_SIGNAL_SOURCE", "Range Table"="rszvl_rngExtGateSource", "Command"="SENS:SWE:EGAT:SOUR", "Read Callback"="", "Write Callback"="", "Range Callback"="", "Check Callback"="", "Rngtable Callback"="", "Coerce Callback"="", "User Callback"="", "Supported Models"="", "Instrument Options"="", "Repeated Capabilities"="", "Restricted Repeated Capabilities"="", "Help"="This attribute toggles between external gate signal and IF power signal as a signal source for the gate mode. If an IF power signal is used, the gate is opened as soon as a signal at > -20 dBm is detected within the IF path bandwidth (50 MHz).\n\nAvailable Repeated Capabilities:\nNone\n\nRemote-control command(s):\n[SENSe<1|2>:]SWEep:EGATe:SOURce EXTernal | IFPower", "Flags"={"OPC Wait"=FALSE, "Dont check status"=FALSE, "*WAI"=FALSE}, "Check Status Callback"=""}, {"Level"=2, "Descriptive Name"="Video Trigger", "Class Only"=TRUE, "Data Type"=0, "Access"=0, "Identifier"="", "Range Table"="", "Command"="", "Read Callback"="", "Write Callback"="", "Range Callback"="", "Check Callback"="", "Rngtable Callback"="", "Coerce Callback"="", "User Callback"="", "Supported Models"="", "Instrument Options"="", "Repeated Capabilities"="", "Restricted Repeated Capabilities"="", "Help"="Attributes to configure and control video triggers.\n\n(1) Video Trigger Level:\nThis attribute sets the level of the video trigger source.", "Flags"={"OPC Wait"=FALSE, "Dont check status"=FALSE, "*WAI"=FALSE}, "Check Status Callback"=""}, {"Level"=3, "Descriptive Name"="Video Trigger Level", "Class Only"=FALSE, "Data Type"=1, "Access"=2, "Identifier"="RSZVL_ATTR_VIDEO_TRIGGER_LEVEL", "Range Table"="rszvl_rngPct", "Command"="TRIG:LEV:VID", "Read Callback"="", "Write Callback"="", "Range Callback"="", "Check Callback"="", "Rngtable Callback"="", "Coerce Callback"="", "User Callback"="", "Supported Models"="", "Instrument Options"="", "Repeated Capabilities"="", "Restricted Repeated Capabilities"="", "Help"="This attribute sets the level of the video trigger source.\n\nAvailable Repeated Capabilities:\nNone\n\nRemote-control command(s):\nTRIGger<1|2>[:SEQuence]:LEVel:VIDeo", "Flags"={"OPC Wait"=FALSE, "Dont check status"=FALSE, "*WAI"=FALSE}, "Check Status Callback"=""}, {"Level"=2, "Descriptive Name"="IF Power Trigger", "Class Only"=TRUE, "Data Type"=0, "Access"=0, "Identifier"="", "Range Table"="", "Command"="", "Read Callback"="", "Write Callback"="", "Range Callback"="", "Check Callback"="", "Rngtable Callback"="", "Coerce Callback"="", "User Callback"="", "Supported Models"="", "Instrument Options"="", "Repeated Capabilities"="", "Restricted Repeated Capabilities"="", "Help"="IF Power Trigger configuration.\n\n(1) Trigger IF Power Level:\nThis attribute sets the level of the IF power trigger source.\n\n(2) Trigger IF Power Offset:\nThis attribute sets the holding time before the next IF power trigger event.\n\n(3) Trigger IF Power Hysteresis:\nThis attribute sets the limit that the hysteresis value has to fall below in order to trigger the next measurement.", "Flags"={"OPC Wait"=FALSE, "Dont check status"=FALSE, "*WAI"=FALSE}, "Check Status Callback"=""}, {"Level"=3, "Descriptive Name"="Trigger IF Power Level", "Class Only"=FALSE, "Data Type"=1, "Access"=2, "Identifier"="RSZVL_ATTR_TRIGGER_IFP_LEVEL", "Range Table"="rszvl_rngTrigIFPowerLevel", "Command"="TRIG:LEV:IFP", "Read Callback"="", "Write Callback"="", "Range Callback"="", "Check Callback"="", "Rngtable Callback"="", "Coerce Callback"="", "User Callback"="", "Supported Models"="", "Instrument Options"="", "Repeated Capabilities"="", "Restricted Repeated Capabilities"="", "Help"="This attribute sets the level of the IF power trigger source.\n\nAvailable Repeated Capabilities:\nNone\n\nRemote-control command(s):\nTRIGger<1|2>[:SEQuence]:LEVel:IFPower", "Flags"={"OPC Wait"=FALSE, "Dont check status"=FALSE, "*WAI"=FALSE}, "Check Status Callback"=""}, {"Level"=3, "Descriptive Name"="Trigger IF Power Offset", "Class Only"=FALSE, "Data Type"=1, "Access"=2, "Identifier"="RSZVL_ATTR_TRIGGER_IFP_OFFSET", "Range Table"="rszvl_rngIFPowOffset", "Command"="TRIG:IFP:HOLD", "Read Callback"="", "Write Callback"="", "Range Callback"="", "Check Callback"="", "Rngtable Callback"="", "Coerce Callback"="", "User Callback"="", "Supported Models"="", "Instrument Options"="", "Repeated Capabilities"="", "Restricted Repeated Capabilities"="", "Help"="This attribute sets the holding time before the next IF power trigger event.\n\nAvailable Repeated Capabilities:\nNone\n\nRemote-control command(s):\nTRIGger<1|2>[:SEQuence]:IFPower:HOLDoff", "Flags"={"OPC Wait"=FALSE, "Dont check status"=FALSE, "*WAI"=FALSE}, "Check Status Callback"=""}, {"Level"=3, "Descriptive Name"="Trigger IF Power Hysteresis", "Class Only"=FALSE, "Data Type"=1, "Access"=2, "Identifier"="RSZVL_ATTR_TRIGGER_IFP_HYSTERESIS", "Range Table"="rszvl_rngIFPowHyst", "Command"="TRIG:IFP:HYST", "Read Callback"="", "Write Callback"="", "Range Callback"="", "Check Callback"="", "Rngtable Callback"="", "Coerce Callback"="", "User Callback"="", "Supported Models"="", "Instrument Options"="", "Repeated Capabilities"="", "Restricted Repeated Capabilities"="", "Help"="This attribute sets the limit that the hysteresis value has to fall below in order to trigger the next measurement.\n\nAvailable Repeated Capabilities:\nNone\n\nRemote-control command(s):\nTRIGger<1|2>[:SEQuence]:IFPower:HYSTeresis", "Flags"={"OPC Wait"=FALSE, "Dont check status"=FALSE, 
